vi "serial read.vi"(8 "error in (no error)":errorcluster, 9 "cnt":i32, 11 "portHandle in":i32) -> (0 "error out":errorcluster, 1 "return value":i32, 2 "data":string, 3 "portHandle out":i32)   [LabVIEW 2016]
uses:
  libc.so.6
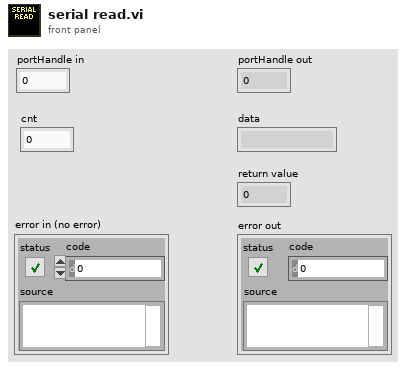
[diagram p1: front panel]
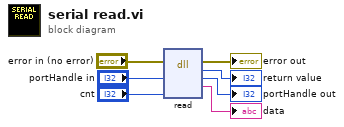
[diagram p0: block diagram]
diagram:
  n1 = dll-call lib="libc.so.6" fn="read"(error in="error in (no error)", "portHandle"="portHandle in", "count"="cnt") -> (error out=→"error out":errorcluster, "return type"=→"return value":i32, "portHandle"=→"portHandle out":i32, "data"=→"data":string)  [unwired: 4 in, 1 out]
